vi "Find MHL Frames.vi"(8 "error in":errorcluster, 10 "Event Name":string, 11 "VI reference":refnum<vi>) -> (0 "error out":errorcluster, 3 "Found?":bool)   [LabVIEW 2020, in "Panther Dashboard.lvlib"]
uses:
  Panther Dashboard.lvlib
  <vilib>/Utility/traverseref.llb/TRef TravTarget.ctl
  <vilib>/Utility/traverseref.llb/VI Scripting - Traverse.lvlib
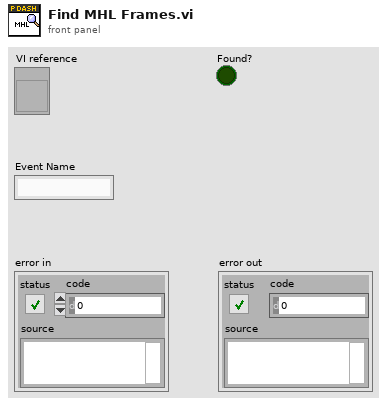
[diagram p1: front panel]
types:
  T1 = typedef "TRef TravTarget.ctl" = enum16{"FP", "BD", "Other"}
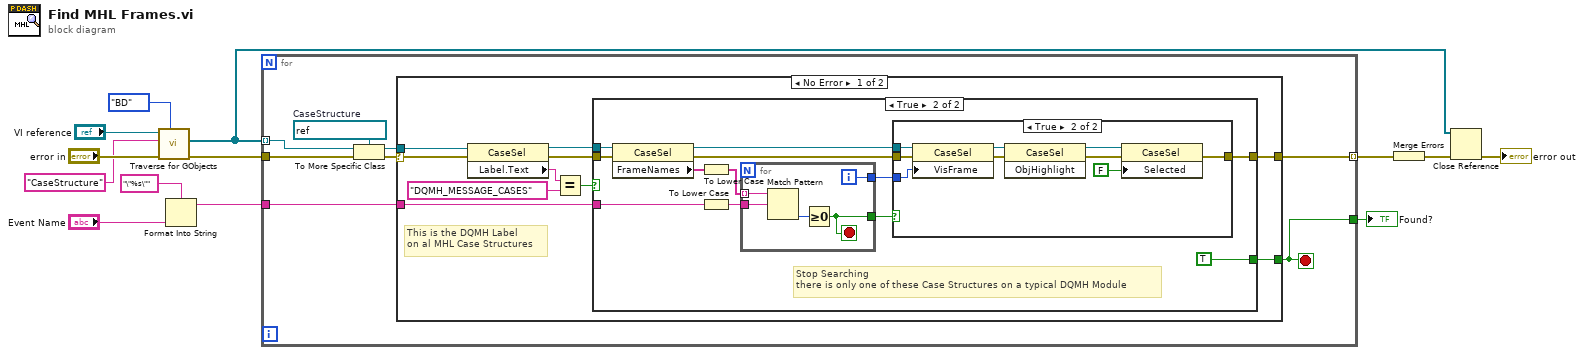
[diagram p0: block diagram]
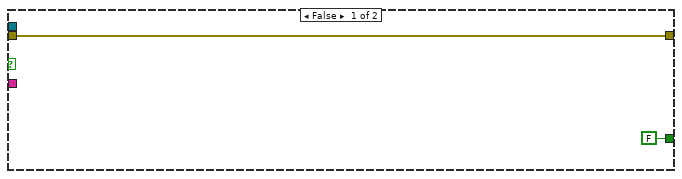
[diagram p2: hidden frame]
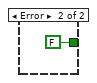
[diagram p4: hidden frame]
diagram:
  n1 = call <vilib>:"Traverse for GObjects.vi"("Traverse Target"=TRef_TravTarget."BD", "error in (no error)"="error in", "Class Name"="CaseStructure", "VI Refnum"="VI reference") -> ("error out"=w11:errorcluster, "References"=w2:refnum<vi>[])  [unwired: 4 in, 2 out]
  n2 = Format Into String(format string="\"%s\"", "Event Name") -> (resulting string=w6:string)  [unwired: 2 in, 1 out]
  n3 = for {
    tunnel: w2 -> [w18] mode=indexing
    tunnel: [w20] -> w9 mode=indexing
    tunnel: w6 -> [w15]
    tunnel: w11 -> [w19]
    tunnel: [w14] -> w1
    stop <- w14 stop-if-true
    w17 = refnum<vi> refnum  # CaseStructure
    n4 = To More Specific Class(target class=w17, reference=w18, error in=w19) -> (specific class reference=w16:refnum<vi>, error out=w21:errorcluster)
    n5 = case shown="No Error" w21 {
      selector: w21 -> [w30 _]
      tunnel: w16 -> [w28 _]
      tunnel: [w31 _] -> w20
      tunnel: w15 -> [w24 _]
      tunnel: [w22 FALSE] -> w14
      frame No Error {
        # "This is the DQMH Label\non al MHL Case Structures"
        n6 = property class="CaseSel"(reference=w28, error in=w30) -> (reference out=w25:refnum<vi>, error out=w29:errorcluster, "Label.Text"=w23:string)
        n7 = Equal?(x=w23, y="DQMH_MESSAGE_CASES") -> (x = y?=w26:bool)
        n8 = case shown="True" w26 {
          tunnel: [w33 w45] -> w31
          tunnel: w25 -> [_ w42]
          tunnel: w24 -> [_ w37]
          tunnel: w29 -> [w33 w44]
          tunnel: [FALSE TRUE] -> w22
          frame False {
          }
          frame True {
            # "Stop Searching\nthere is only one of these Case Structures on a typical DQMH Module"
            n9 = property class="CaseSel"(reference=w42, error in=w44) -> (reference out=w39:refnum<vi>, error out=w43:errorcluster, "FrameNames"=w41:string[])
            n10 = To Lower Case(string=w41) -> (all lower case string=w35:string[])
            n11 = To Lower Case(string=w37) -> (all lower case string=w36:string)
            n12 = for {
              tunnel: w35 -> [w56] mode=indexing
              tunnel: w36 -> [w59]
              tunnel: [w60] -> w40
              tunnel: [w57] -> w38
              i -> [w60]
              stop <- w57 stop-if-true
              n13 = Match Pattern(string=w56, regular expression=w59) -> (offset past match=w58:i32)  [unwired: 1 in, 3 out]
              n14 = Greater Or Equal To 0?(x=w58) -> (x >= 0?=w57:bool)
            }
            n15 = case shown="True" w38 {
              tunnel: [w46 w52] -> w45
              tunnel: w43 -> [w46 w53]
              tunnel: w40 -> [_ w50]
              tunnel: w39 -> [_ w49]
              frame False {
              }
              frame True {
                n16 = property class="CaseSel"(reference=w49, error in=w53, "VisFrame"=w50) -> (reference out=w51:refnum<vi>, error out=w55:errorcluster)
                n17 = invoke class="CaseSel" method="ObjHighlight"(reference=w51, error in=w55) -> (reference out=w48:refnum<vi>, error out=w54:errorcluster)  [unwired: 1 in, 1 out]
                n18 = property class="CaseSel"(reference=w48, error in=w54, "Selected"=FALSE) -> (error out=w52:errorcluster)  [unwired: 1 out]
              }
            }
          }
        }
      }
      frame Error {
      }
    }
  }
  "Found?" <- w1
  n19 = Merge Errors(w9) -> (w12:errorcluster)
  n20 = Close Reference(reference=w2, error in (no error)=w12) -> (error out=→"error out":errorcluster)
